vi "Connection Reference.vi"(7 "action":enum16{"Write", "Read"}(ring)=enum."Read", 11 "connection ID in":refnum<k5>) -> (3 "connection ID out":refnum<k5>)   [LabVIEW 2015]
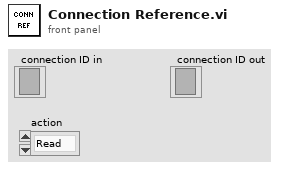
[diagram p1: front panel]
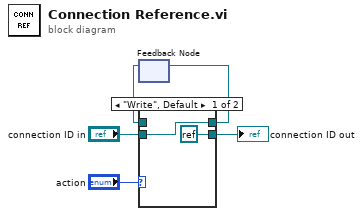
[diagram p0: block diagram]
diagram:
  n1 = feedback #1() -> (w3:refnum<k5>)  [unwired: 1 in]
  n2 = case shown="\"Write\", Default" "action" {
    tunnel: "connection ID in" -> [w7 _]
    tunnel: [w7 w8] -> w4
    tunnel: [refnum<k0> refnum w8] -> w1
    tunnel: w3 -> [_ w8]
    frame "Write", Default {
    }
    frame "Read" {
    }
  }
  "connection ID out" <- w1
  n3 = feedback-in #1(w4) -> ()
